vi "remote.Read Sys.PhysChanProperties.vi"(8 "error in (no error)":errorcluster, 11 "SLSC Remote in":refnum<class "SLSC Remote.lvclass">) -> (0 "error out":errorcluster, 2 "Sys.PhysChanProperties":refnum<k21>[](array[refnum]), 3 "SLSC Remote out":refnum<class "SLSC Remote.lvclass">)   [LabVIEW 2016, in "SLSC Interfaces.lvlib" / "SLSC Remote.lvclass"]
uses:
  SLSC Remote.lvclass
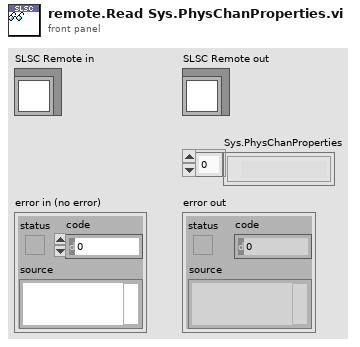
[diagram p1: front panel]
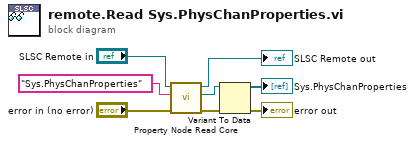
[diagram p0: block diagram]
diagram:
  n1 = call "Property Node Read Core.vi"("error in (no error)"="error in (no error)", "property"="Sys.PhysChanProperties", "SLSC Remote in"="SLSC Remote in") -> ("error out"=w8:errorcluster, "value"=w3:refnum<class "JSON Null.lvclass">, "SLSC Remote out"=→"SLSC Remote out":refnum<class "SLSC Remote.lvclass">)  [unwired: 6 in]
  n2 = Variant To Data(error in=w8, Variant=w3) -> (data=→"Sys.PhysChanProperties":refnum<k21>[], error out=→"error out":errorcluster)  [unwired: 1 in]
